vi "Filter String, Pass Floating Point.vi"(1 "Input String":string) -> (0 "Numeric String":string)   [LabVIEW 2020]
doc: "Remove all characters except: 0-9, plus, minus, and decimal point."
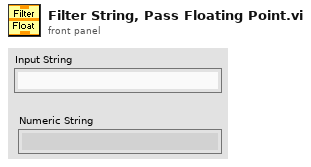
[diagram p1: front panel]
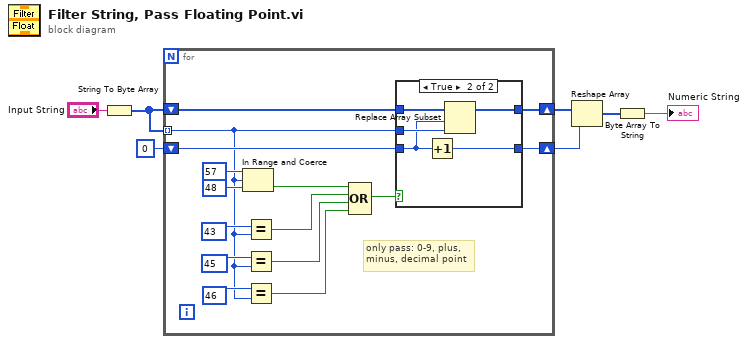
[diagram p0: block diagram]
diagram:
  n1 = String To Byte Array(string="Input String") -> (unsigned byte array=w5:u8[])
  n2 = for {
    tunnel: w5 -> [w8] mode=indexing
    shift-right: [w20] -> w1
    shift-left: 0 ("lower limit") -> [w19]
    shift-right: [w18] -> w4
    shift-left: w5 -> [w17]
    # "only pass: 0-9, plus, minus, decimal point"
    n3 = In Range and Coerce(upper limit=u8 57, x=w8, lower limit=u8 48) -> (In Range?=w15:bool)  [unwired: 1 out]
    n4 = Equal?(x=u8 43 ("lower limit"), y=w8) -> (x = y?=w11:bool)
    n5 = Equal?(x=u8 45 ("lower limit"), y=w8) -> (x = y?=w10:bool)
    n6 = Equal?(x=u8 46 ("lower limit"), y=w8) -> (x = y?=w9:bool)
    n7 = Compound Arithmetic op=OR(w15, w11, w10, w9) -> (w16:bool)
    n8 = case shown="True" w16 {
      tunnel: [w24 w29] -> w20
      tunnel: w19 -> [w24 w25]
      tunnel: [w23 w28] -> w18
      tunnel: w17 -> [w23 w27]
      tunnel: w8 -> [_ w26]
      frame False {
      }
      frame True {
        n9 = Increment(x=w25) -> (x+1=w29:i32)
        n10 = Replace Array Subset(array=w27, new element=w26, index=w25) -> (w28:u8[])
      }
    }
  }
  n11 = Reshape Array(w4, w1) -> (w3:u8[])
  n12 = Byte Array To String(unsigned byte array=w3) -> (string=→"Numeric String":string)
